vi "find tag by name.vi"(10 "name":string, 11 "tags in":refnum<class "tag descriptor.lvclass">[](array[class])) -> (3 "index":i32)   [LabVIEW 2013, in "tag bus.lvlib" / "tag descriptor.lvclass"]
doc: "Locates a specific tag by name in the provided list of tags."
uses:
  tag descriptor.lvclass
  tag descriptor.lvclass/tag descriptor.ctl
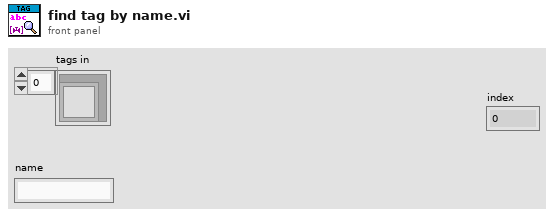
[diagram p1: front panel]
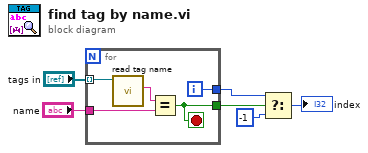
[diagram p0: block diagram]
diagram:
  n1 = for {
    tunnel: "tags in" -> [w11] mode=indexing
    tunnel: "name" -> [w9]
    tunnel: [w8] -> w4
    tunnel: [w7] -> w3
    i -> [w7]
    stop <- w8 stop-if-true
    n2 = call "read tag name.vi"("system tag in"=w11) -> ("name"=w10:string)  [unwired: 8 in, 2 out]
    n3 = Equal?(x=w10, y=w9) -> (x = y?=w8:bool)
  }
  n4 = Select(t=w3, s=w4, f=-1) -> (s? t:f=→"index":i32)
